vi "Load Data.vi"(8 "error in (no error)":errorcluster caption="错误输入（无错误）") -> (0 "error out":errorcluster caption="错误输出", 3 "New Graph Data":waveform(dbl)[](array[waveform]) caption="新图形数据")   [LabVIEW 2013]
doc: "从磁盘的文件加载数据。"
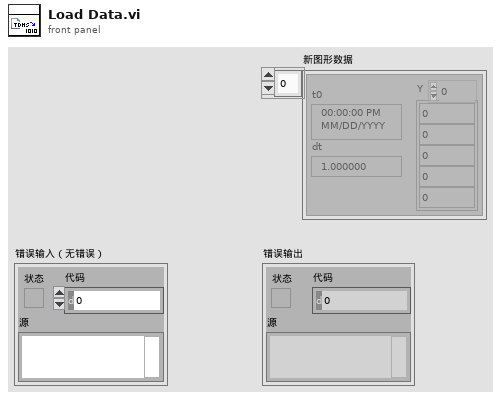
[diagram p1: front panel]
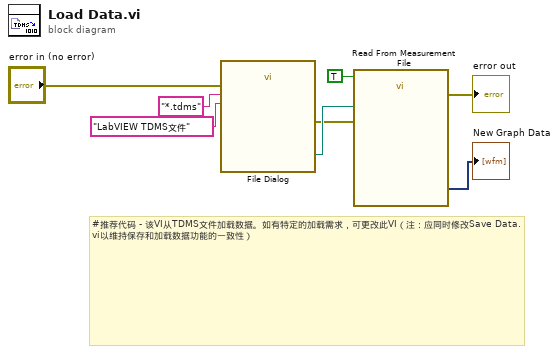
[diagram p0: block diagram]
diagram:
  # "#推荐代码 - 该VI从TDMS文件加载数据。如有特定的加载需求，可更改此VI（注：应同时修改Save Data.vi以维持保存和加载数据功能的一致性）"
  n1 = call "File Dialog"("error in"="error in (no error)", "pattern (all files)"="*.tdms", "pattern label"="LabVIEW TDMS文件" ("LabVIEW TDMS File")) -> ("selected path"=w2:path, "error out"=w1:errorcluster)  [unwired: 9 in, 2 out]
  n2 = call "Read From Measurement File"("error in (no error)"=w1, "Filename"=w2, "Reset"=TRUE) -> ("error out"=→"error out":errorcluster, "Signals"=→"New Graph Data":dynamicdata)  [unwired: 3 in, 4 out]
